vi "Read Draw Toolbar Event.vi"(8 "error in (no error)":errorcluster, 11 "Toolbar Control in":refnum<class "Toolbar Control.lvclass">) -> (0 "error out":errorcluster, 2 "Draw Toolbar Event":refnum<user-event>, 3 "Toolbar Control out":refnum<class "Toolbar Control.lvclass">)   [LabVIEW 2011, in "Toolbar Control.lvclass"]
doc: "-------------\nDeveloped by Brian Hoover (hooovahh)"
uses:
  Toolbar Control.lvclass
  Toolbar Control.lvclass/Toolbar Control.ctl
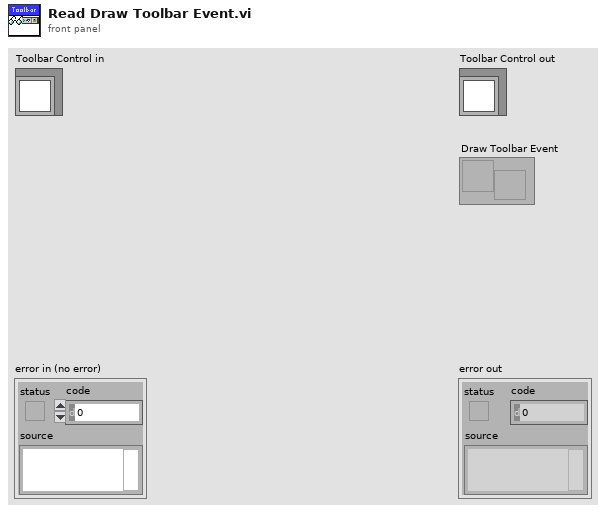
[diagram p1: front panel]
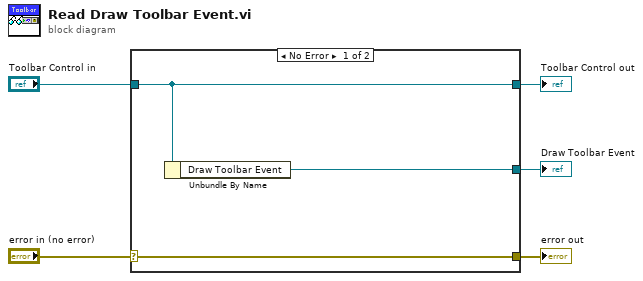
[diagram p0: block diagram]
diagram:
  n1 = case shown="No Error" "error in (no error)" {
    selector: "error in (no error)" -> [w8 w9]
    tunnel: [w8 w9] -> w4
    tunnel: [w7 w10] -> w2
    tunnel: "Toolbar Control in" -> [w7 w10]
    tunnel: [w6 _] -> w1
    frame No Error {
      n2 = Unbundle By Name(w7) -> ("Draw Toolbar Event"=w6:refnum<user-event>)
    }
    frame Error {
    }
  }
  "error out" <- w4
  "Toolbar Control out" <- w2
  "Draw Toolbar Event" <- w1
